vi "readbuffer.vi"(8 "error in (no error)":errorcluster, 11 "MSCU":refnum<class "MSCU.lvclass">) -> (0 "error out":errorcluster, 2 "Buffer":string, 3 "MSCU":refnum<class "MSCU.lvclass">)   [LabVIEW 2019, in "MSCU.lvclass"]
uses:
  MSCU.lvclass
  MSCU.lvclass/MSCU.ctl
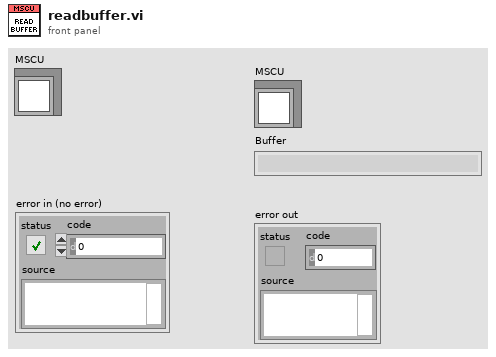
[diagram p1: front panel]
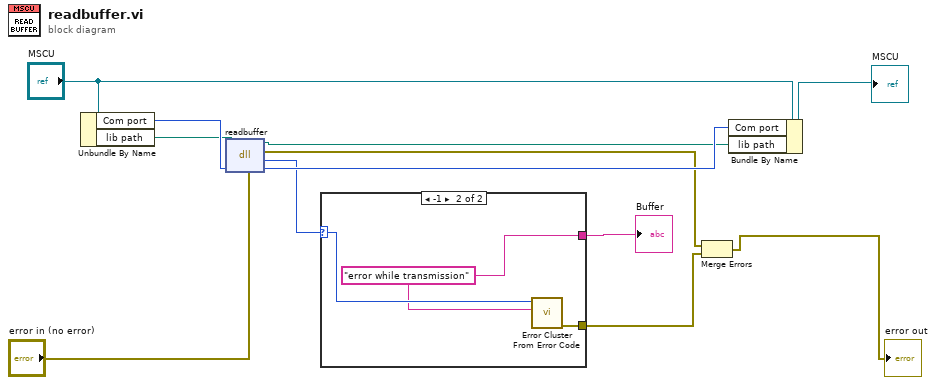
[diagram p0: block diagram]
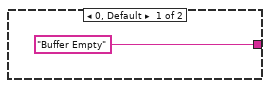
[diagram p2: hidden frame]
diagram:
  n1 = Unbundle By Name("MSCU") -> ("Com port"=w5:i32, "lib path"=w4:path)
  n2 = dll-call lib="C:/Program Files (x86)/Nanonis/SPM Controller/data/MSCU.dll" fn="readbuffer"(path in=w4, error in="error in (no error)", "Comport"=w5) -> (path out=w2:path, error out=w10:errorcluster, "return type"=w8:i32, "Comport"=w11:i32)  [unwired: 1 in]
  n3 = case shown="-1" w8 {
    selector: w8 -> [_ w16]
    tunnel: ["Buffer Empty" w14] -> w9
    tunnel: [_ w15] -> w12
    frame 0, Default {
    }
    frame -1 {
      w14 = "error while transmission"
      n4 = call <vilib>:"Error Cluster From Error Code.vi"("error message (\"\")"=w14, "error code (0)"=w16) -> ("error out"=w15:errorcluster)  [unwired: 7 in]
    }
  }
  "Buffer" <- w9
  n5 = Merge Errors(w10, w12) -> (→"error out":errorcluster)
  n6 = Bundle By Name(cluster="MSCU", "Com port"=w11, "lib path"=w2) -> (→"MSCU":refnum<class "MSCU.lvclass">)
